vi "Read from Text File.vi"() -> ()   [LabVIEW 2015]
doc: "This example shows how the Write to Text File and Read from Text File functions operate using different options."
panel:
  out "array":i32[](array[numeric])
  out "rnx":i32
  in  "threshold":i32=3
  out "Bit Sequence":dbl[](array[numeric]) format="%#.6g"
  in  "basepath":path=path "D:/Users/Documents/LabVIEW Data/FeryRFID_VI/rfid_vi/RN16_learn/trial03"
  out "appended path":path
  out "Read Text":string="\n"
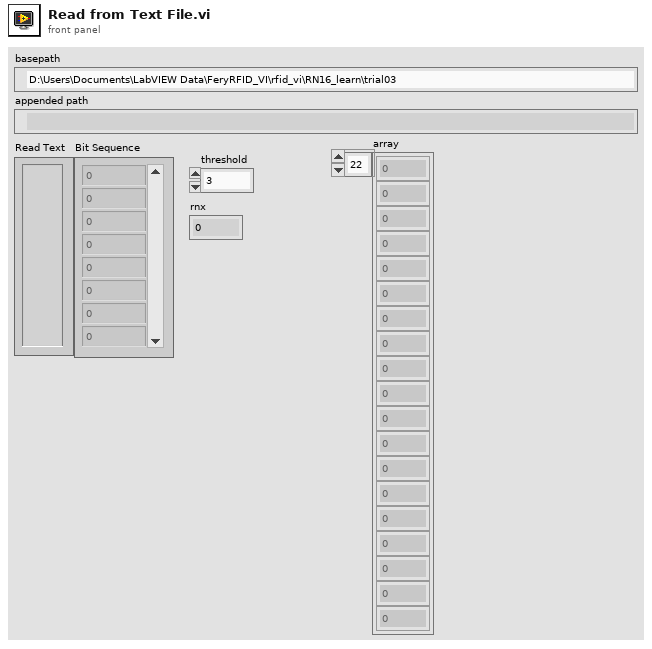
[diagram p1: front panel]
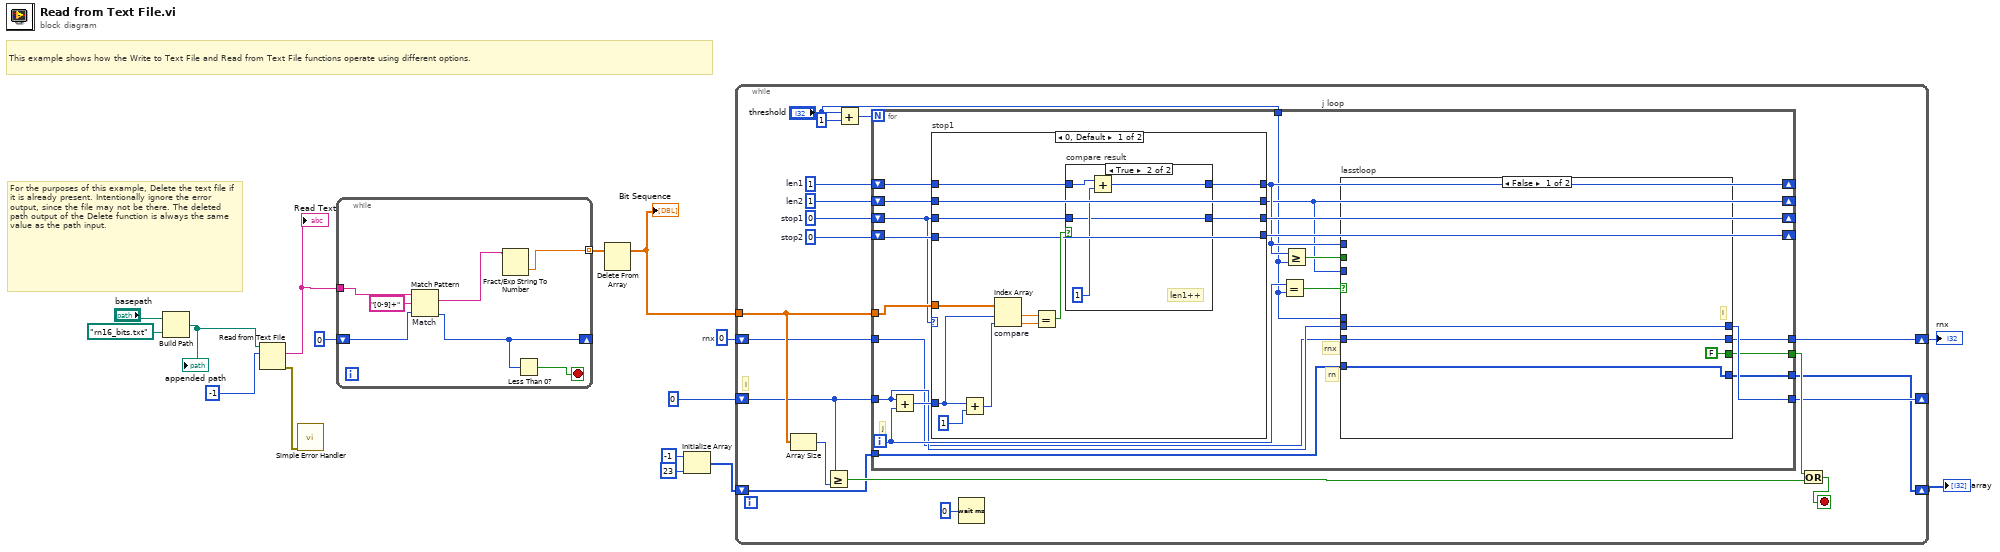
[diagram p0: block diagram]
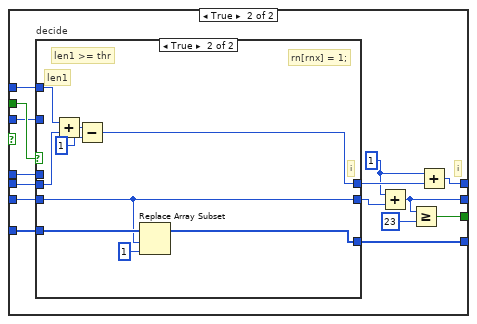
[diagram p2: hidden frame]
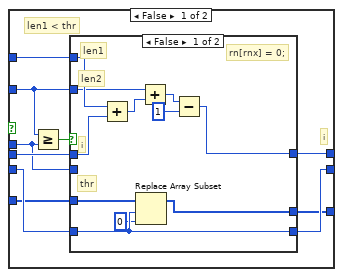
[diagram p3: hidden frame]
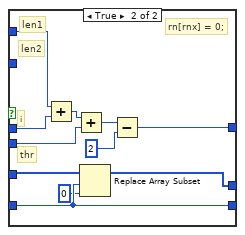
[diagram p4: hidden frame]
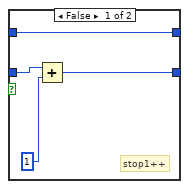
[diagram p5: hidden frame]
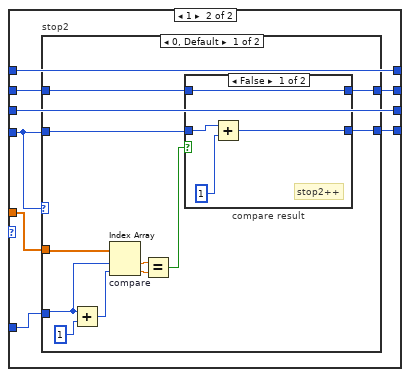
[diagram p6: hidden frame]
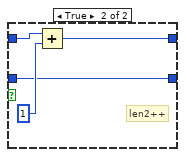
[diagram p7: hidden frame]
diagram:
  w6 = 0  # rnx
  # "This example shows how the Write to Text File and Read from Text File functions operate using different options."
  # "For the purposes of this example, Delete the text file if it is already present. Intentionally ignore the error output, since the file may not be there. The deleted path output of the Delete function is always the same value as the path input."
  n1 = Build Path(base path="basepath", name or relative path=path "rn16_bits.txt" ("default name")) -> (appended path=w13:path)
  "appended path" <- w13
  n2 = Read from Text File(file (use dialog)=w13, count=-1) -> (text=w11:string, error out=w14:errorcluster)  [unwired: 2 in, 2 out]
  "Read Text" <- w11
  n3 = call <vilib>:"Simple Error Handler.vi"("error in (no error)"=w14) -> ()  [unwired: 4 in, 5 out]
  n4 = while {
    tunnel: w11 -> [w23]
    shift-right: [w18] -> _
    shift-left: 0 -> [w22]
    tunnel: [w20] -> w9 mode=indexing
    stop <- w19 stop-if-true
    n5 = Match Pattern "Match"(string=w23, regular expression="[0-9]+", offset (0)=w22) -> (match substring=w21:string, offset past match=w18:i32)  [unwired: 2 out]
    n6 = Fract/Exp String To Number(string=w21) -> (number=w20:dbl)  [unwired: 3 in, 1 out]
    n7 = Less Than 0?(x=w18) -> (x < 0?=w19:bool)
  }
  n8 = Delete From Array(array=w9) -> (array with subset deleted=w8:dbl[])  [unwired: 2 in, 1 out]
  "Bit Sequence" <- w8
  n9 = Initialize Array(-1 ("element"), 23 ("dimension size")) -> (w4:i32[])
  n10 = while {
    tunnel: w8 -> [w38]
    shift-right: [w26] -> _
    shift-left: 0 -> [w27]
    shift-right: [w29] -> w7
    shift-left: w6 -> [w28]
    shift-right: [w24] -> w1
    shift-left: w4 -> [w25]
    stop <- w35 stop-if-true
    w42 = 0  # stop2
    w41 = 0  # stop1
    w40 = 1  # len2
    w39 = 1  # len1
    # "i"
    n11 = Array Size(array=w38) -> (size(s)=w37:i32)
    n12 = Greater Or Equal?(x=w27, y=w37) -> (x >= y?=w34:bool)
    n13 = Add(x="threshold", y=1) -> (x+y=w31:i32)
    n14 = for "j loop" {
      N: w31 -> [_]
      tunnel: w38 -> [w59]
      shift-right: [w51] -> _
      shift-left: w39 -> [w63]
      shift-right: [w57] -> _
      shift-left: w41 -> [w58]
      shift-right: [w56] -> _
      shift-left: w42 -> [w61]
      shift-right: [w47] -> _
      shift-left: w40 -> [w62]
      tunnel: "threshold" -> [w45]
      tunnel: [w46] -> w36
      tunnel: w27 -> [w52]
      tunnel: [w50] -> w26
      tunnel: w28 -> [w49]
      tunnel: [w48] -> w29
      tunnel: w25 -> [w44]
      tunnel: [w43] -> w24
      i -> [w55]
      # "rn"
      # "rnx"
      # "j"
      n15 = Add(x=w52, y=w55) -> (x+y=w60:i32)
      n16 = case "stop1" shown="0, Default" w58 {
        tunnel: w63 -> [w129 w152]
        tunnel: w62 -> [w125 w147]
        tunnel: w61 -> [w124 w149]
        tunnel: w60 -> [w135 w145]
        tunnel: w59 -> [w133 w150]
        tunnel: [w128 w152] -> w51
        tunnel: w58 -> [w127 w151]
        tunnel: [w126 w151] -> w57
        tunnel: [w124 w148] -> w56
        tunnel: [w125 w146] -> w47
        frame 0, Default {
          n17 = Add(x=w135, y=1) -> (x+y=w136:i32)
          n18 = Index Array "compare"(array=w133, index #1=w135, index #2=w136) -> (element #1=w131:dbl, element #2=w132:dbl)
          n19 = Equal?(x=w131, y=w132) -> (x = y?=w130:bool)
          n20 = case "compare result" shown="True" w130 {
            tunnel: w129 -> [w140 w144]
            tunnel: [w140 w143] -> w128
            tunnel: w127 -> [w138 w141]
            tunnel: [w139 w141] -> w126
            frame False {
              # "stop1++"
              n21 = Add(x=w138, y=1) -> (x+y=w139:i32)
            }
            frame True {
              # "len1++"
              n22 = Add(x=w144, y=1) -> (x+y=w143:i32)
            }
          }
        }
        frame 1 {
          n23 = case "stop2" shown="0, Default" w149 {
            tunnel: w150 -> [w160 _]
            tunnel: w149 -> [w159 w172]
            tunnel: [w158 w172] -> w148
            tunnel: w147 -> [w157 w173]
            tunnel: [w156 w173] -> w146
            tunnel: w145 -> [w153 _]
            frame 0, Default {
              n24 = Add(x=w153, y=1) -> (x+y=w161:i32)
              n25 = Index Array "compare"(array=w160, index #1=w153, index #2=w161) -> (element #1=w163:dbl, element #2=w162:dbl)
              n26 = Equal?(x=w163, y=w162) -> (x = y?=w154:bool)
              n27 = case "compare result" shown="False" w154 {
                tunnel: w157 -> [w167 w171]
                tunnel: [w167 w170] -> w156
                tunnel: w159 -> [w165 w168]
                tunnel: [w166 w168] -> w158
                frame False {
                  # "stop2++"
                  n28 = Add(x=w165, y=1) -> (x+y=w166:i32)
                }
                frame True {
                  # "len2++"
                  n29 = Add(x=w171, y=1) -> (x+y=w170:i32)
                }
              }
            }
            frame 1 {
            }
          }
        }
      }
      n30 = Equal?(x=w55, y=w45) -> (x = y?=w54:bool)
      n31 = Greater Or Equal?(x=w51, y=w45) -> (x >= y?=w53:bool)
      n32 = case "lasstloop" shown="False" w54 {
        tunnel: w53 -> [_ w80]
        tunnel: w52 -> [w67 w82]
        tunnel: w51 -> [_ w81]
        tunnel: [w67 w73] -> w50
        tunnel: w49 -> [w66 w71]
        tunnel: [w66 w78] -> w48
        tunnel: w47 -> [_ w79]
        tunnel: [FALSE w76] -> w46
        tunnel: w45 -> [_ w75]
        tunnel: w44 -> [w64 w69]
        tunnel: [w64 w68] -> w43
        frame False {
          # "i"
        }
        frame True {
          w72 = 1 ("y")
          # "i"
          n33 = case "decide" shown="True" w80 {
            tunnel: w82 -> [w92 w122]
            tunnel: w81 -> [w88 w123]
            tunnel: [w87 w120] -> w74
            tunnel: w79 -> [w90 _]
            tunnel: w75 -> [w89 _]
            tunnel: [w85 w116] -> w70
            tunnel: w71 -> [w86 w116]
            tunnel: w69 -> [w84 w118]
            tunnel: [w83 w117] -> w68
            frame False {
              # "i"
              # "len1 < thr"
              n34 = Greater Or Equal?(x=w90, y=w89) -> (x >= y?=w91:bool)
              n35 = case shown="False" w91 {
                tunnel: w90 -> [w100 _]
                tunnel: w92 -> [w102 w113]
                tunnel: w89 -> [_ w111]
                tunnel: w88 -> [w103 w114]
                tunnel: [w97 w108] -> w87
                tunnel: [w95 w105] -> w85
                tunnel: w86 -> [w95 w105]
                tunnel: w84 -> [w96 w107]
                tunnel: [w93 w106] -> w83
                frame False {
                  # "rn[rnx] = 0;"
                  # "thr"
                  # "len2"
                  # "i"
                  # "len1"
                  n36 = Add(x=w103, y=w102) -> (x+y=w101:i32)
                  n37 = Replace Array Subset(array=w96, new element=0 ("new element/subarray"), index=w95) -> (w93:i32[])
                  n38 = Add(x=w100, y=w101) -> (x+y=w99:i32)
                  n39 = Subtract(x=w99, y=1) -> (x-y=w97:i32)
                }
                frame True {
                  # "rn[rnx] = 0;"
                  # "len2"
                  # "thr"
                  # "i"
                  # "len1"
                  n40 = Add(x=w114, y=w113) -> (x+y=w112:i32)
                  n41 = Add(x=w112, y=w111) -> (x+y=w110:i32)
                  n42 = Replace Array Subset(array=w107, new element=0 ("new element/subarray"), index=w105) -> (w106:i32[])
                  n43 = Subtract(x=w110, y=2) -> (x-y=w108:i32)
                }
              }
            }
            frame True {
              # "rn[rnx] = 1;"
              # "len1"
              # "i"
              # "len1 >= thr"
              n44 = Add(x=w123, y=w122) -> (x+y=w121:i32)
              n45 = Subtract(x=w121, y=1) -> (x-y=w120:i32)
              n46 = Replace Array Subset(array=w118, new element=1 ("new element/subarray"), index=w116) -> (w117:i32[])
            }
          }
          n47 = Add(x=w72, y=w70) -> (x+y=w78:i32)
          n48 = Greater Or Equal?(x=w78, y=23) -> (x >= y?=w76:bool)
          n49 = Add(x=w72, y=w74) -> (x+y=w73:i32)
        }
      }
    }
    n50 = Wait (ms)(milliseconds to wait=u32 0) -> ()  [unwired: 1 out]
    n51 = Or(x=w36, y=w34) -> (x .or. y?=w35:bool)
  }
  "rnx" <- w7
  "array" <- w1
